vi "Main Monitor Loop.vi"(8 "error in (no error)":errorcluster, 11 "main ref":T1) -> (0 "error out":errorcluster)   [LabVIEW 2025]
uses:
  controls/LAB-IQ UI Data.ctl
panel:
  out "Test Stop Temp":bool
  out "DepthZ":dbl
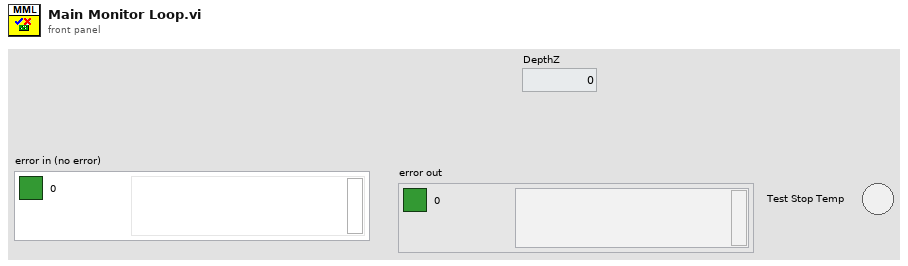
[diagram p1: front panel]
types:
  T1 = typedef "LAB-IQ UI Data.ctl" = cluster{"Main Home Screen":cluster{"GUI":refnum<vi>, "Platform Settings":refnum<vi>, "Configure":refnum<vi>, "Home":refnum<vi>, "EXIT":refnum<vi>, "service 2":refnum<vi>, "MainPage":refnum<vi>, "Analysis":refnum<vi>}, "Platform Settings":cluster{"mm/s  Surge":refnum<vi>, "Update Surge Speed":refnum<vi>, "Drive Error":refnum<vi>, "Disable Axis Jog Soft Limits":refnum<vi>, "mm/s  Sway":refnum<vi>, "Sway and Surge COM Status":refnum<vi>, "Heave COM Status":refnum<vi>, "Enable Platform":refnum<vi>, "Surge Forward Main":refnum<vi>, "Sway Right Main":refnum<vi>, "Sway Left Main":refnum<vi>, "Heave Down Main":refnum<vi>, "Heave Up main":refnum<vi>, "Update Sway Speed":refnum<vi>, "Update Heave Speed":refnum<vi>, "mm/s Heave":refnum<vi>, "mm/sec":refnum<vi>, "mm":refnum<vi>, "Surge Backward Main":refnum<vi>}, "Analysis Screen":cluster{"Analysis Home":refnum<vi>, "Surface Analysis":refnum<vi>, "Imaging":refnum<vi>, "Image Analysis":refnum<vi>, "Post Analysis":refnum<vi>}, "Config Screen":cluster{"Select Load Head":refnum<vi>, "Notes :":refnum<vi>, "FILE":refnum<vi>, "Sample ID :":refnum<vi>, "Operator ID :":refnum<vi>, "Operator Name :":refnum<vi>, "Auto":refnum<vi>}, "Motion Module":cluster{"zNL":refnum<vi>, "NL disp":refnum<vi>, "Rotary Tab":refnum<vi>, "Motion Direction:  3":refnum<vi>, "E.Velocity 2":refnum<vi>, "e.v/ssr 2":refnum<vi>, "Enter Fixed E.Velocity 2":refnum<vi>, "Enter Final SRR 2":refnum<vi>, "Enter initial SRR 2":refnum<vi>, "Enter Fixed SRR 2":refnum<vi>, "Enter the Final E.Velocity (m/s) 2":refnum<vi>, "Enter initial E.Velocity (m/s) 2":refnum<vi>, "Final Speed (RPM) 3":refnum<vi>, "Initial Speed (RPM) 2":refnum<vi>, "Enter the Final Velocity (m/s) 3":refnum<vi>, "Enter initial Velocity (m/s)  3":refnum<vi>, "Ramp Up 2":refnum<vi>, "TEST SELECTION":refnum<vi>, "SPEED SELECTION : ":refnum<vi>, "Angular Oscillation Set":refnum<vi>, "Traction":refnum<vi>, "Step Speed":refnum<vi>, "StepTable For Load-Speed":refnum<vi>, "StepTable For Speed":refnum<vi>, "Surge Forward MM":refnum<vi>, "Surge Backward MM":refnum<vi>, "M3 Image":refnum<vi>, "String 39":refnum<vi>, "Sway Left MM":refnum<vi>, "Sway Right MM":refnum<vi>, "Disable Axis Jog Soft Limits":refnum<vi>, "mm":refnum<vi>, "Heave Down MM":refnum<vi>, "Heave Up MM":refnum<vi>, "Wear Track Diameter (mm)":refnum<vi>, "Set WTD":refnum<vi>, "HomeScratch":refnum<vi>, "HomeRot":refnum<vi>, "PlaceModule":refnum<vi>, "Enter the Angle (Deg)":refnum<vi>, "Enter the Frequency (Hz)":refnum<vi>, "Motion Mode:":refnum<vi>, "LR Sway":refnum<vi>, "Rot Hor":refnum<vi>, "Scratch":refnum<vi>, "LR Cam":refnum<vi>, "MMBack":refnum<vi>, "MMNext":refnum<vi>, "Rot Ver":refnum<vi>, "Rotary Module Selection":refnum<vi>, "calculate rotary":refnum<vi>, "SPEED SELECTION : rotary":refnum<vi>, "Import 2":refnum<vi>, "Save 2":refnum<vi>, "File Path :  2":refnum<vi>, "String 45":refnum<vi>, "StepTable For Speed 3":refnum<vi>, "Enter the Speed(mm/sec)":refnum<vi>, "Enter the Speed(RPM)":refnum<vi>, "Enter Scratch Speed (mm/s):":refnum<vi>, "SwaySpeed Set":refnum<vi>, "Scartch Offset":refnum<vi>, "Motion type:":refnum<vi>, "HomeScratch 2":refnum<vi>, "Enter Scratch length (mm):":refnum<vi>, "Wear Track Diameter":refnum<vi>, "Rotary Speed Exced":refnum<vi>, "Scratch Mode":refnum<vi>, "No of Scratch":refnum<vi>}, "Environmental control":cluster{"Humidity  Status  3":refnum<vi>, "Low Temp  Status  2":refnum<vi>, "TK4 status 2":refnum<vi>, "Stage Temperature":refnum<vi>, "Sample Temperature":refnum<vi>, "Humidity (Amb)":refnum<vi>, "Clear List":refnum<vi>, "Add to list":refnum<vi>, "Wear":refnum<vi>, "Vibration":refnum<vi>, "Humidity (Chamber)":refnum<vi>, "Temperature (Chamber)":refnum<vi>, "ECR ":refnum<vi>, "Temperature (Amb)":refnum<vi>, "Microphone":refnum<vi>, "Acoustic Emission 3":refnum<vi>, "SNext":refnum<vi>, "APBack":refnum<vi>, "Enter the Temperature (°C):":refnum<vi>, "Enter the Stage \nTemperature (°C):":refnum<vi>, "Enter the Humidity (%Rh):":refnum<vi>, "Low Temp":refnum<vi>, "High Temp":refnum<vi>, "Humidity":refnum<vi>, "Sensors Picked":refnum<vi>}, "About Screen":cluster{"Password":refnum<vi>, "Home Service":refnum<vi>, "Advanced Setting":refnum<vi>, "About Tab":refnum<vi>, "ECR Port:":refnum<vi>, "Ramp Port:":refnum<vi>, "Installation/Replacement completed":refnum<vi>, "Loahead":refnum<vi>, "Heave and Surge COM Port:":refnum<vi>, "Sway COM Port:":refnum<vi>, "Temp Modbus:":refnum<vi>, "Humidity Port:":refnum<vi>, "Edit Gain Constants":refnum<vi>, "Save Gain Constants":refnum<vi>}, "Main Screen":cluster{"Main Screen Tab":refnum<vi>, "Angle and Frequency":refnum<vi>, "Stroke (mm)":refnum<vi>, "Angle (Deg)":refnum<vi>, "Main Speed Tab":refnum<vi>, "MTM MOTOR DISPLAY":refnum<vi>, "Disc Speed (m/sec)":refnum<vi>, "Ball Speed (m/sec)":refnum<vi>, "Disc Speed (RPM)":refnum<vi>, "Ball Speed (RPM)":refnum<vi>, "SPEED TAB":refnum<vi>, "Speed (m/sec)":refnum<vi>, "Set Speed (m/sec)":refnum<vi>, "Speed (RPM)":refnum<vi>, "Set Speed":refnum<vi>, "Time Tab":refnum<vi>, "Time ( HH:MM:SS ) 2":refnum<vi>, "Test Duration":refnum<vi>, "Test Duration 4":refnum<vi>, "TEST CYCLE":refnum<vi>, "TOTAL CYCLES":refnum<vi>, "Set Load (N)":refnum<vi>, "Temp Tabs":refnum<vi>, "Heater":refnum<vi>, "TK4 status":refnum<vi>, "ChamberTemp":refnum<vi>, "SetTmp":refnum<vi>, "Controller  Status":refnum<vi>, "ChamberTemp 2":refnum<vi>, "SetTmp 2":refnum<vi>, "Controller  Status 2":refnum<vi>, "ChamberTemp 3":refnum<vi>, "SetTmp 3":refnum<vi>, "Cooling":refnum<vi>, "Load Communication":refnum<vi>, "Ambient \nTemperature":refnum<vi>, "HumCOMStatus":refnum<vi>, "Ambient\n Humidity":refnum<vi>, "Freq (Hz)":refnum<vi>, "Load En":refnum<vi>, "NLt":refnum<vi>, "zNL 2":refnum<vi>, "Humidity On":refnum<vi>, "humidity disp":refnum<vi>, "Set Humidity":refnum<vi>, "NL disp 2":refnum<vi>, "Humidity On 2":refnum<vi>, "humidity disp 2":refnum<vi>, "Set Humidity 2":refnum<vi>, "NL disp 3":refnum<vi>, "AppLoadSeq scratch":refnum<vi>, "Stop Scratch":refnum<vi>, "ClrLog":refnum<vi>, "Trip Log":refnum<vi>, "STOP":refnum<vi>, "Start Test":refnum<vi>, "Test status":refnum<vi>, "AR Led":refnum<vi>, "Data":refnum<vi>, "Health":refnum<vi>, "Sway COM Status":refnum<vi>, "Heave COM Status":refnum<vi>, "Grp Tab":refnum<vi>, "Sub Graph":refnum<vi>, "SD (mm)":refnum<vi>, "Siliding distance Reset Graph":refnum<vi>, "SDGp":refnum<vi>, "Humidity Reset Graph":refnum<vi>, "HumrGp":refnum<vi>, "Acoustic Emission (mV)":refnum<vi>, "Aqucostic Reset Graph":refnum<vi>, "gACQUOS":refnum<vi>, "ECR RESET":refnum<vi>, "ECR":refnum<vi>, "Temperature Reset":refnum<vi>, "Acoustic Emission (mV) 2":refnum<vi>, "Aqucostic Reset Graph 2":refnum<vi>, "gACQUOS 2":refnum<vi>, "ECR RESET 2":refnum<vi>, "ECR 2":refnum<vi>, "Temperature Reset 2":refnum<vi>, "Temperature (deg c)":refnum<vi>, "Speed Reset Graph":refnum<vi>, "Speed Tab":refnum<vi>, "MTM DISC  SPEED":refnum<vi>, "MTM BALL SPEED":refnum<vi>, "speed mm/sec":refnum<vi>, "Hymidity":refnum<vi>, "Humidity Disable trip":refnum<vi>, "CoF Trip  2":refnum<vi>, "Depth Trip":refnum<vi>, "Weart Deapth":refnum<vi>, "Depth Reset Graph":refnum<vi>, "Weart":refnum<vi>, "Depthz":refnum<vi>, "Depth (µm)":refnum<vi>, "WearGp":refnum<vi>, "NL Trip 2":refnum<vi>, "Load pid":refnum<vi>, "Load Disable Trip":refnum<vi>, "Load Reset Graph":refnum<vi>, "NL Display 4":refnum<vi>, "Main Chart 3":refnum<vi>, "BACK":refnum<vi>, "Depth Trip 2":refnum<vi>, "COF TRIP ":refnum<vi>, "Friction Force (N)":refnum<vi>, "FF Reset Graph":refnum<vi>, "FF Disable Trip":refnum<vi>, "FF TRIP":refnum<vi>, "COF Disable Trip":refnum<vi>, "COF Reset Graph":refnum<vi>, "Start Test Temp":refnum<vi>, "zFF":refnum<vi>, "Friction Force (N) Graph":refnum<vi>, "Coefficient of Friction":refnum<vi>, "Scratch Start Test":refnum<vi>, "FF Tab":refnum<vi>, "Cyclic Friction Force (N)":refnum<vi>, "CZ FF":refnum<vi>, "Cyclic Friction Force (N) Graph":refnum<vi>, "Cyclic Coefficient of Friction":refnum<vi>, "Cyclic FF TRIP":refnum<vi>, "Cyclic FF Disable Trip":refnum<vi>, "cyclic COF Disable Trip":refnum<vi>, "cyclic COF TRIP":refnum<vi>, "cyclic COF Reset Graph":refnum<vi>, "Cyclic FF Reset Graph":refnum<vi>, "Test Trip":refnum<vi>, "Multi Scratch Pass":refnum<vi>, "Scratch Start Recording":refnum<vi>}, "Loading":cluster{"Indentation":refnum<vi>, "Reference Sample":refnum<vi>, "Load Cell Communication Slide":refnum<vi>, "com 3":refnum<vi>, "com":refnum<vi>, "DecaForce COM Status":refnum<vi>, "Update":refnum<vi>, "Clear 3":refnum<vi>, "seq":refnum<vi>, "Stribeck table":refnum<vi>, "Stribeck Table  For loading":refnum<vi>, "Loading Mode":refnum<vi>, "Enter the Final Load (N)":refnum<vi>, "Enter the CoF Trip":refnum<vi>, "Enter the Friction Force Trip":refnum<vi>, "Enter the Normal load Trip":refnum<vi>, "Enter the Load  (N)":refnum<vi>, "KiloForce":refnum<vi>, "DecaForce ":refnum<vi>, "MicroForce":refnum<vi>, "LHBack":refnum<vi>, "LHNext":refnum<vi>, "Enter the Loading Rate (N/min)":refnum<vi>, "Message":refnum<vi>, "Warning 2":refnum<vi>, "SSP 0.75":refnum<vi>, "SSP 0.5":refnum<vi>, "SSP 0.3":refnum<vi>, "Warning":refnum<vi>, "gui GIF":refnum<vi>, "Communication is established":refnum<vi>, "AppLoad 4":refnum<vi>, "Multipoint":refnum<vi>, "Load Selection":refnum<vi>}, "PID":cluster{"Ramp MulFac":refnum<vi>, "pulses LoadDiffRamp(2..10)":refnum<vi>, "PulseControlRamp(diff<=3N)":refnum<vi>, "SetLoadDeadband(%) Load(0-10N)":refnum<vi>, "PID gains out delay (microForce)":refnum<vi>, "Ramp":refnum<vi>, "Gain 2":refnum<vi>, "pulses LoadDiff(2..10)":refnum<vi>, "pulses LoadDiff(11..50)":refnum<vi>, "PulseControl(diff<=3N)":refnum<vi>, "SetLoadDeadband(%)  2":refnum<vi>, "Dummy Run":refnum<vi>, "Vertical load (N)":refnum<vi>, "AutoTune":refnum<vi>, "Offset 3 ":refnum<vi>, "apply load":refnum<vi>, "Offset  3":refnum<vi>, "apply load 2":refnum<vi>, "Enter ByPass Load":refnum<vi>, "reinit 3":refnum<vi>, "output range delay":refnum<vi>, "PID gains out delay":refnum<vi>, "Bypass Load":refnum<vi>, "pulsesSent":refnum<vi>, "pulses ":refnum<vi>, "actpid":refnum<vi>, "gFF Rot":refnum<vi>, "pulses LoadDiff(21..1000)":refnum<vi>, "Delay":refnum<vi>, "deadband":refnum<vi>}, "Config Parameters":cluster{"Tab Control 3":refnum<vi>, "Tab Control 19":refnum<vi>, "SAMPLES":refnum<vi>, "Re-initilaize":refnum<vi>, "Filter ON/OFF":refnum<vi>, "TracHomeSurgeOffsetCounts 10MM":refnum<vi>, "TracHomeSwayOffsetCounts 10MM":refnum<vi>, "Acoustic Emission:":refnum<vi>, "Apply Filter (FF)":refnum<vi>, "Filter% 2":refnum<vi>, "Apply Filter (Load)":refnum<vi>, "Filter% ":refnum<vi>, "Sway distance (mm)":refnum<vi>, "Surge distance (mm)":refnum<vi>, "DataSavingLoopDelay(ms)":refnum<vi>, "SAVE 2":refnum<vi>, "Enter Distance":refnum<vi>, "Sway Counts:":refnum<vi>, "Distance (mm): 3":refnum<vi>, "Surge Counts:":refnum<vi>, "Distance (mm): 2":refnum<vi>, "Distance (mm):":refnum<vi>, "Heave Counts:":refnum<vi>, "LRMHomeSurgeOffsetCounts":refnum<vi>, "LRMHomeSwayOffsetCounts":refnum<vi>, "TracHomeSurgeOffsetCounts 20MM":refnum<vi>, "TracHomeSwayOffsetCounts 20MM":refnum<vi>, "RotHomeSwayOffsetCounts":refnum<vi>, "RotHomeSurgeOffsetCounts":refnum<vi>, "Heave distance":refnum<vi>, "Zmm":refnum<vi>, "Heave Pulses/mm":refnum<vi>, "Surge Pulses/mm":refnum<vi>, "Sway Pulses/mm":refnum<vi>, "Heave Pitch":refnum<vi>, "Surge Pitch":refnum<vi>, "Sway Pitch":refnum<vi>, "Heave PPR":refnum<vi>, "Surge PPR":refnum<vi>, "Sway PPR":refnum<vi>, "Tab Control 5":refnum<vi>, "Tab Control 14":refnum<vi>, "Tab Control 26":refnum<vi>, "AE":refnum<vi>, "Heave Loop Delay":refnum<vi>, "Heave PID Speed":refnum<vi>, "Surge Jog Speed":refnum<vi>, "Heave Jog Speed":refnum<vi>, "Sway Loop Delay":refnum<vi>, "Sway PID Speed":refnum<vi>, "Sway Jog Speed":refnum<vi>, "DEPTH TRIP VALUE":refnum<vi>, "LOAD TRIP VALUE":refnum<vi>, "DEPTH TRIP   ENABLE":refnum<vi>, "LOAD TRIP  ENABLE":refnum<vi>, "CYCLIC FF TRIP VALUE":refnum<vi>, "FF TRIP VALUE":refnum<vi>, "CYCLIC CoF TRIP VALUE":refnum<vi>, "COF TRIP VALUE":refnum<vi>, "CYCLIC COF TRIP  ENABLE":refnum<vi>, "CYCLIC FF TRIP  ENABLE":refnum<vi>, "FF TRIP  ENABLE":refnum<vi>, "COF TRIP  ENABLE":refnum<vi>}, "Loading Com Port":cluster{"ClearAll":refnum<vi>, "Mz(Nm)":refnum<vi>, "My(Nm)":refnum<vi>, "Mx(Nm)":refnum<vi>, "Save Dwell":refnum<vi>, "Mx ":refnum<vi>, "My ":refnum<vi>, "Mz":refnum<vi>, "Fx(N)":refnum<vi>, "Fy(N)":refnum<vi>, "Fz(N)":refnum<vi>, "ZeroAll":refnum<vi>, "Acq Delay (ms)":refnum<vi>, "Burst Delay (ms)":refnum<vi>, "model":refnum<vi>, "SN":refnum<vi>, "FFx(N)":refnum<vi>, "Sensor IP":refnum<vi>, "Port":refnum<vi>, "FFy(N)":refnum<vi>, "Load(N)":refnum<vi>, "delete Handle":refnum<vi>, "Create Handle":refnum<vi>, "ft_data":refnum<vi>, "ft_range":refnum<vi>, "ft_data 2":refnum<vi>, "stop 6":refnum<vi>, "running_flag":refnum<vi>, "ft_udp_handle":refnum<vi>, "get-data-return":refnum<vi>, "get-range-return":refnum<vi>, "zero-return":refnum<vi>, "filter-return":refnum<vi>, "initial-return":refnum<vi>, "deleteHandle-result":refnum<vi>, "Load Cell Temp":refnum<vi>}, "Heave AND Surge":cluster{"SURGE POSE":refnum<vi>, "error out Read":refnum<vi>, "HEAVE POSE":refnum<vi>, "State":refnum<vi>, "Homed":refnum<vi>, "Sequence ID":refnum<vi>, "error out Write":refnum<vi>, "faultCode":refnum<vi>, "Ack ID":refnum<vi>, "SPEED":refnum<vi>, "Distance":refnum<vi>, "Mode Command":refnum<vi>, "Heave and Surge Read":refnum<vi>, "Read Heave Temp":refnum<vi>, "Spare 15":refnum<vi>, "Spare 14":refnum<vi>, "Spare 13":refnum<vi>, "Spare 12":refnum<vi>, "Spare 11":refnum<vi>, "Spare 10":refnum<vi>, "Spare 9":refnum<vi>, "Spare 8":refnum<vi>, "Spare 7":refnum<vi>, "Spare 6":refnum<vi>, "Spare 5":refnum<vi>, "Spare 4":refnum<vi>, "Spare 2":refnum<vi>, "Spare 1":refnum<vi>, "Node Id":refnum<vi>, "Spare 3":refnum<vi>, "SPARE 4":refnum<vi>, "SPARE 3":refnum<vi>, "SPARE 2":refnum<vi>, "SPARE 1":refnum<vi>, "fwMajor":refnum<vi>, "fwMinor":refnum<vi>, "Manual Write":refnum<vi>, "Heave and Surge Write":refnum<vi>}, "New PID LOGIC":cluster{"Fine Tune Zone":refnum<vi>, "PID SDelay":refnum<vi>, "Max_pos_limit":refnum<vi>, "Min_pos_limit":refnum<vi>, "i_limit":refnum<vi>, "pct_scale":refnum<vi>, "Deadband":refnum<vi>, "Kd":refnum<vi>, "Ki":refnum<vi>, "Kp":refnum<vi>, "Current Position":refnum<vi>, "Set Load":refnum<vi>, "Current Load":refnum<vi>, "Pulse delta":refnum<vi>, "Init Step":refnum<vi>, "Max Step Linit":refnum<vi>}, "SWAY ":cluster{"fwMajor":refnum<vi>, "Homed":refnum<vi>, "Rotary POSE":refnum<vi>, "State":refnum<vi>, "SWAY POSE":refnum<vi>, "Ack ID":refnum<vi>, "faultCode":refnum<vi>, "Node Id":refnum<vi>, "fwMinor":refnum<vi>, "Spare 6":refnum<vi>, "Spare 5":refnum<vi>, "Spare 4":refnum<vi>, "Spare 3":refnum<vi>, "Spare 2":refnum<vi>, "Spare 1":refnum<vi>, "Spare 7":refnum<vi>, "SPARE  5":refnum<vi>, "error out Write  SWAY ":refnum<vi>, "error out Read SWAY ":refnum<vi>, "Manual Write SWAY ":refnum<vi>, "SWAY WRITE":refnum<vi>, "SPARE  4":refnum<vi>, "SPARE  3":refnum<vi>, "SPARE 2":refnum<vi>, "SPARE 1":refnum<vi>, "Spare 15":refnum<vi>, "Spare 14":refnum<vi>, "Spare 13":refnum<vi>, "Spare 12":refnum<vi>, "Spare 11":refnum<vi>, "Spare 9":refnum<vi>, "Spare 8":refnum<vi>, "SPEED":refnum<vi>, "Distance":refnum<vi>, "Mode Command":refnum<vi>, "Sequence ID":refnum<vi>, "SWAY READ":refnum<vi>, "Spare 10":refnum<vi>, "Read SWAY Temp":refnum<vi>}, "Analysis Screen":cluster{"Analysis Home":refnum<vi>, "Refresh 2":refnum<vi>, "MEAN 4":refnum<vi>, "SD 4":refnum<vi>, "VARIANCE 4":refnum<vi>, "MEAN  3":refnum<vi>, "SD  3":refnum<vi>, "VARIANCE  3":refnum<vi>, "MEAN 2":refnum<vi>, "SD  2":refnum<vi>, "VARIANCE 2":refnum<vi>, "MEAN":refnum<vi>, "SD":refnum<vi>, "VARIANCE":refnum<vi>, "File 4 Discription":refnum<vi>, "OPEN 4":refnum<vi>, "File Name 4":refnum<vi>, "OPEN 3":refnum<vi>, "File 3 Discription":refnum<vi>, "File Name 3":refnum<vi>, "Y-AXIS":refnum<vi>, "X-AXIS":refnum<vi>, "XY Graph":refnum<vi>, "File Name 2":refnum<vi>, "File Name 1":refnum<vi>, "OPEN 2":refnum<vi>, "OPEN 1":refnum<vi>, "File 1 Discription ":refnum<vi>, "File 2 Discription":refnum<vi>, "Export":refnum<vi>, "File Format":refnum<vi>}}
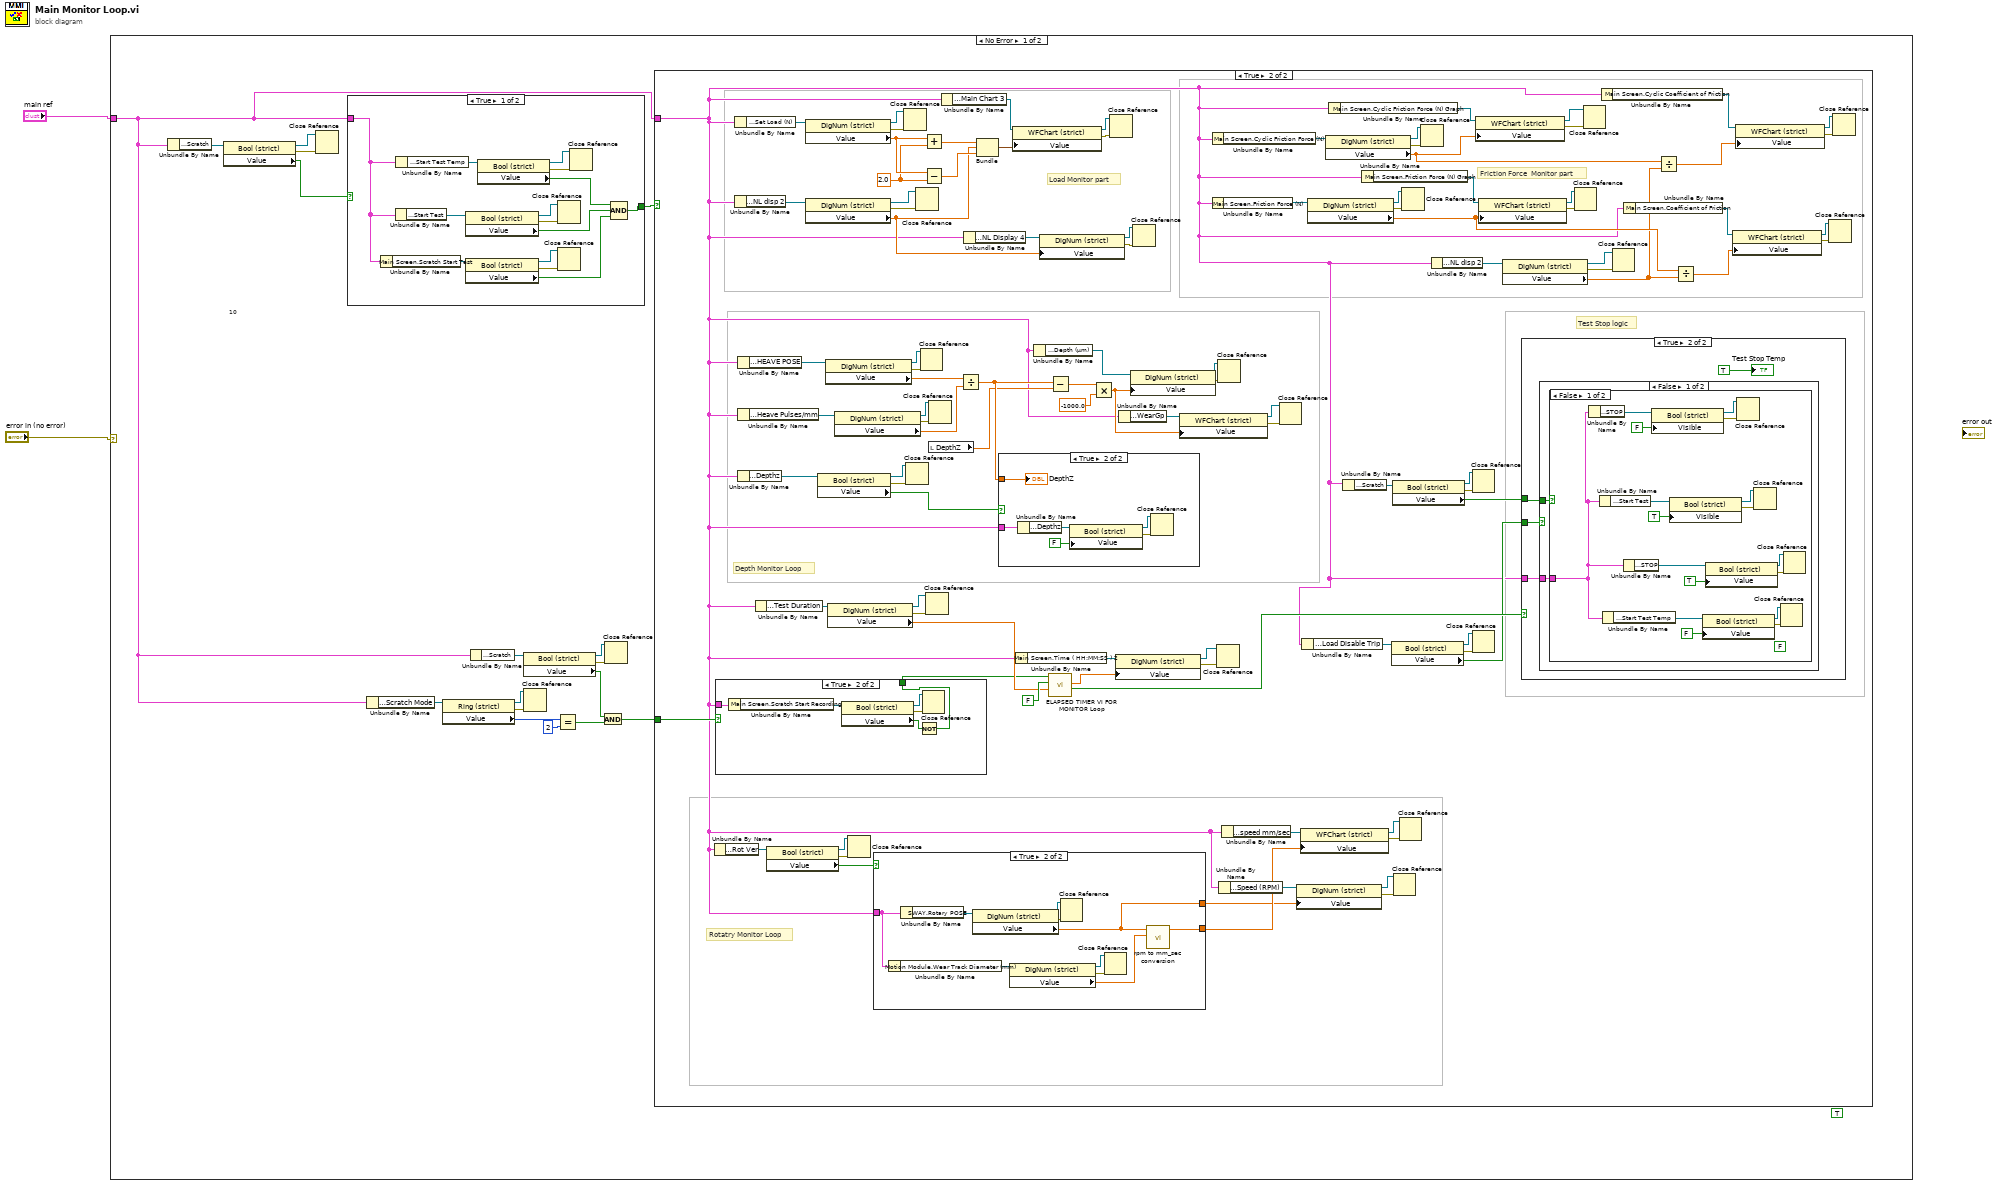
[diagram p0: block diagram]
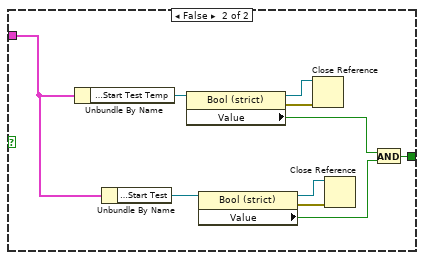
[diagram p2: hidden frame]
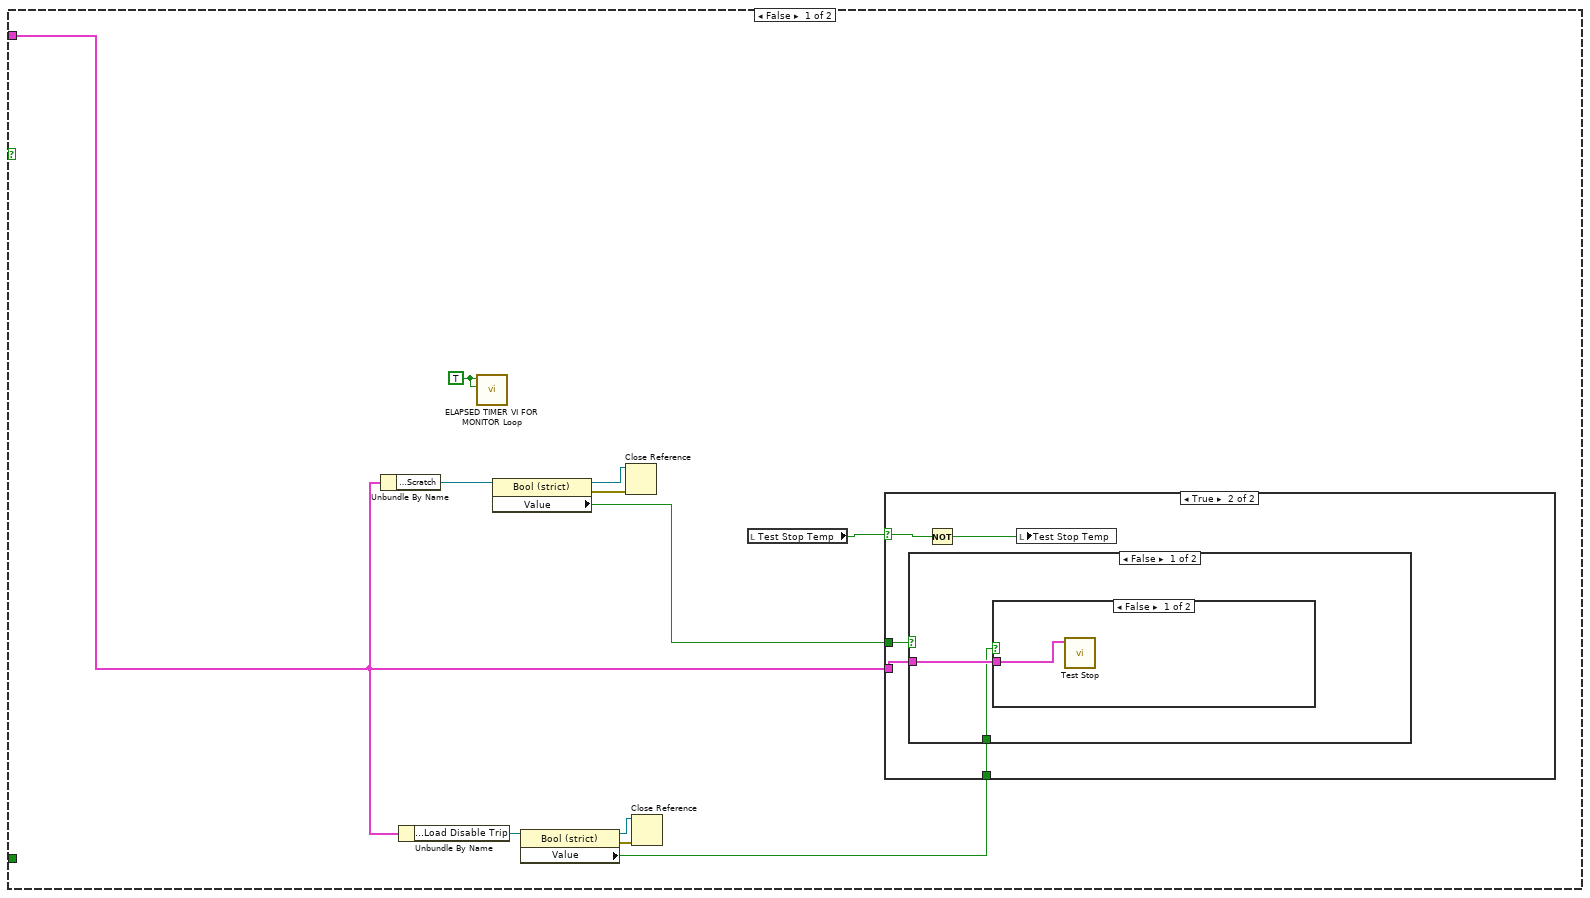
[diagram p3: hidden frame]
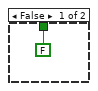
[diagram p7: hidden frame]
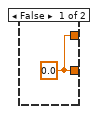
[diagram p8: hidden frame]
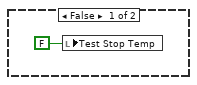
[diagram p9: hidden frame]
diagram:
  n1 = case shown="No Error" "error in (no error)" {
    tunnel: "main ref" -> [w6 _]
    frame No Error {
      (unwired) TRUE
      # "10"
      n2 = Unbundle By Name(w6) -> ("Motion Module.Scratch"=w17:refnum<vi>)
      n3 = property class="Bool (strict)"(reference=w17) -> (reference out=w18:refnum<vi>, error out=w16:errorcluster, "Value"=w15:bool)  [unwired: 1 in]
      n4 = Close Reference(reference=w18, error in (no error)=w16) -> ()  [unwired: 1 out]
      n5 = case shown="True" w15 {
        tunnel: w6 -> [w21 w37]
        tunnel: [w25 w35] -> w19
        frame True {
          n6 = Unbundle By Name(w21) -> ("Main Screen.Scratch Start Test"=w23:refnum<vi>)
          n7 = Unbundle By Name(w21) -> ("Main Screen.Start Test"=w29:refnum<vi>)
          n8 = Unbundle By Name(w21) -> ("Main Screen.Start Test Temp"=w32:refnum<vi>)
          n9 = property class="Bool (strict)"(reference=w29) -> (reference out=w28:refnum<vi>, error out=w30:errorcluster, "Value"=w26:bool)  [unwired: 1 in]
          n10 = property class="Bool (strict)"(reference=w23) -> (reference out=w24:refnum<vi>, error out=w22:errorcluster, "Value"=w20:bool)  [unwired: 1 in]
          n11 = property class="Bool (strict)"(reference=w32) -> (reference out=w33:refnum<vi>, error out=w31:errorcluster, "Value"=w27:bool)  [unwired: 1 in]
          n12 = Close Reference(reference=w28, error in (no error)=w30) -> ()  [unwired: 1 out]
          n13 = Close Reference(reference=w24, error in (no error)=w22) -> ()  [unwired: 1 out]
          n14 = Close Reference(reference=w33, error in (no error)=w31) -> ()  [unwired: 1 out]
          n15 = Compound Arithmetic op=AND(w27, w26, w20) -> (w25:bool)
        }
        frame False {
          n16 = Unbundle By Name(w37) -> ("Main Screen.Start Test Temp"=w42:refnum<vi>)
          n17 = Unbundle By Name(w37) -> ("Main Screen.Start Test"=w39:refnum<vi>)
          n18 = property class="Bool (strict)"(reference=w42) -> (reference out=w43:refnum<vi>, error out=w41:errorcluster, "Value"=w36:bool)  [unwired: 1 in]
          n19 = property class="Bool (strict)"(reference=w39) -> (reference out=w38:refnum<vi>, error out=w40:errorcluster, "Value"=w34:bool)  [unwired: 1 in]
          n20 = Close Reference(reference=w43, error in (no error)=w41) -> ()  [unwired: 1 out]
          n21 = Close Reference(reference=w38, error in (no error)=w40) -> ()  [unwired: 1 out]
          n22 = And(x=w36, y=w34) -> (x .and. y?=w35:bool)
        }
      }
      n23 = Unbundle By Name(w6) -> ("Motion Module.Scratch Mode"=w10:refnum<vi>)
      n24 = property class="Ring (strict)"(reference=w10) -> (reference out=w11:refnum<vi>, error out=w9:errorcluster, "Value"=w8:u16)  [unwired: 1 in]
      n25 = Unbundle By Name(w6) -> ("Motion Module.Scratch"=w13:refnum<vi>)
      n26 = property class="Bool (strict)"(reference=w13) -> (reference out=w12:refnum<vi>, error out=w14:errorcluster, "Value"=w4:bool)  [unwired: 1 in]
      n27 = Close Reference(reference=w11, error in (no error)=w9) -> ()  [unwired: 1 out]
      n28 = Equal?(x=w8, y=u16 2) -> (x = y?=w5:bool)
      n29 = And(x=w4, y=w5) -> (x .and. y?=w3:bool)
      n30 = Close Reference(reference=w12, error in (no error)=w14) -> ()  [unwired: 1 out]
      n31 = case shown="True" w19 {
        tunnel: w6 -> [w45 w64]
        tunnel: w3 -> [_ w65]
        frame False {
          w54 = TRUE ("PAUSE")
          n32 = Unbundle By Name(w45) -> ("Motion Module.Scratch"=w52:refnum<vi>)
          n33 = Unbundle By Name(w45) -> ("Main Screen.Load Disable Trip"=w46:refnum<vi>)
          n34 = call "ELAPSED TIMER VI FOR MONITOR Loop.vi"("RESET"=w54, "PAUSE"=w54) -> ()  [unwired: 7 in, 3 out]
          n35 = property class="Bool (strict)"(reference=w52) -> (reference out=w50:refnum<vi>, error out=w51:errorcluster, "Value"=w49:bool)  [unwired: 1 in]
          n36 = property class="Bool (strict)"(reference=w46) -> (reference out=w48:refnum<vi>, error out=w47:errorcluster, "Value"=w44:bool)  [unwired: 1 in]
          n37 = Close Reference(reference=w50, error in (no error)=w51) -> ()  [unwired: 1 out]
          n38 = Close Reference(reference=w48, error in (no error)=w47) -> ()  [unwired: 1 out]
          n39 = local read "Test Stop Temp"() -> (w53:bool)
          n40 = case shown="True" w53 {
            selector: w53 -> [_ w59]
            tunnel: w45 -> [_ w57]
            tunnel: w49 -> [_ w56]
            tunnel: w44 -> [_ w55]
            frame False {
            }
            frame True {
              n41 = case shown="False" w56 {
                tunnel: w57 -> [w61 _]
                tunnel: w55 -> [w60 _]
                frame False {
                  n42 = case shown="False" w60 {
                    tunnel: w61 -> [w62 _]
                    frame False {
                      n43 = call "Test Stop.vi"("Data Cluster"=w62) -> ()  [unwired: 10 in, 1 out]
                    }
                    frame True {
                    }
                  }
                }
                frame True {
                }
              }
              n44 = Not(x=w59) -> (.not. x?=w58:bool)
              n45 = local write "Test Stop Temp"(w58) -> ()
            }
          }
        }
        frame True {
          w150 = 2.0 ("y")
          # "Rotatry Monitor Loop"
          # "Test Stop logic"
          # "Depth Monitor Loop"
          # "Friction Force  Monitor part"
          # "Load Monitor part"
          n46 = Unbundle By Name(w64) -> ("Motion Module.Rot Ver"=w81:refnum<vi>)
          n47 = case shown="True" w65 {
            tunnel: w64 -> [_ w166]
            tunnel: [FALSE ("Value") w164] -> w63
            frame False {
            }
            frame True {
              n48 = Unbundle By Name(w166) -> ("Main Screen.Scratch Start Recording"=w168:refnum<vi>)
              n49 = property class="Bool (strict)"(reference=w168) -> (reference out=w167:refnum<vi>, error out=w169:errorcluster, "Value"=w165:bool)  [unwired: 1 in]
              n50 = Not(x=w165) -> (.not. x?=w164:bool)
              n51 = Close Reference(reference=w167, error in (no error)=w169) -> ()  [unwired: 1 out]
            }
          }
          n52 = Unbundle By Name(w64) -> ("Main Screen.Set Load (N)"=w152:refnum<vi>)
          n53 = Unbundle By Name(w64) -> ("Main Screen.NL disp 2"=w162:refnum<vi>)
          n54 = Unbundle By Name(w64) -> ("Heave AND Surge.HEAVE POSE"=w144:refnum<vi>)
          n55 = Unbundle By Name(w64) -> ("Config Parameters.Heave Pulses/mm"=w141:refnum<vi>)
          n56 = Unbundle By Name(w64) -> ("Main Screen.Depthz"=w136:refnum<vi>)
          n57 = Unbundle By Name(w64) -> ("Main Screen.Test Duration"=w120:refnum<vi>)
          n58 = property class="Bool (strict)"(reference=w81) -> (reference out=w79:refnum<vi>, error out=w80:errorcluster, "Value"=w78:bool)  [unwired: 1 in]
          n59 = property class="DigNum (strict)"(reference=w152) -> (reference out=w146:refnum<vi>, error out=w153:errorcluster, "Value"=w151:dbl)  [unwired: 1 in]
          n60 = property class="DigNum (strict)"(reference=w162) -> (reference out=w160:refnum<vi>, error out=w161:errorcluster, "Value"=w97:dbl)  [unwired: 1 in]
          n61 = property class="Bool (strict)"(reference=w136) -> (reference out=w137:refnum<vi>, error out=w135:errorcluster, "Value"=w134:bool)  [unwired: 1 in]
          n62 = property class="DigNum (strict)"(reference=w144) -> (reference out=w145:refnum<vi>, error out=w143:errorcluster, "Value"=w139:sgl)  [unwired: 1 in]
          n63 = property class="DigNum (strict)"(reference=w120) -> (reference out=w121:refnum<vi>, error out=w119:errorcluster, "Value"=w118:dbl)  [unwired: 1 in]
          n64 = property class="DigNum (strict)"(reference=w141) -> (reference out=w140:refnum<vi>, error out=w142:errorcluster, "Value"=w138:dbl)  [unwired: 1 in]
          n65 = Close Reference(reference=w79, error in (no error)=w80) -> ()  [unwired: 1 out]
          n66 = case shown="True" w78 {
            tunnel: w64 -> [_ w174]
            tunnel: [w170 w172] -> w74
            tunnel: [w170 w171] -> w70
            frame False {
              w170 = 0.0 ("Enter initial Velocity (m/s)  4")
            }
            frame True {
              n67 = Unbundle By Name(w174) -> ("Motion Module.Wear Track Diameter (mm)"=w177:refnum<vi>)
              n68 = Unbundle By Name(w174) -> ("SWAY.Rotary POSE"=w178:refnum<vi>)
              n69 = property class="DigNum (strict)"(reference=w178) -> (reference out=w180:refnum<vi>, error out=w179:errorcluster, "Value"=w171:sgl)  [unwired: 1 in]
              n70 = property class="DigNum (strict)"(reference=w177) -> (reference out=w175:refnum<vi>, error out=w176:errorcluster, "Value"=w173:dbl)  [unwired: 1 in]
              n71 = Close Reference(reference=w180, error in (no error)=w179) -> ()  [unwired: 1 out]
              n72 = Close Reference(reference=w175, error in (no error)=w176) -> ()  [unwired: 1 out]
              n73 = call "rpm to mm_sec conversion.vi"("Wear Track Diameter"=w173, "Initial Speed (RPM)"=w171) -> ("Enter initial Velocity (m/s)  4"=w172:dbl)  [unwired: 7 in, 2 out]
            }
          }
          n74 = Close Reference(reference=w146, error in (no error)=w153) -> ()  [unwired: 1 out]
          n75 = Close Reference(reference=w137, error in (no error)=w135) -> ()  [unwired: 1 out]
          n76 = Close Reference(reference=w160, error in (no error)=w161) -> ()  [unwired: 1 out]
          n77 = Close Reference(reference=w145, error in (no error)=w143) -> ()  [unwired: 1 out]
          n78 = Add(x=w151, y=w150) -> (x+y=w149:dbl)
          n79 = Subtract(x=w151, y=w150) -> (x-y=w148:dbl)
          n80 = Close Reference(reference=w121, error in (no error)=w119) -> ()  [unwired: 1 out]
          n81 = Close Reference(reference=w140, error in (no error)=w142) -> ()  [unwired: 1 out]
          n82 = local read "DepthZ"() -> (w132:dbl)
          n83 = Unbundle By Name(w64) -> ("Main Screen.Main Chart 3"=w156:refnum<vi>)
          n84 = Divide(x=w139, y=w138) -> (x/y=w133:dbl)
          n85 = Unbundle By Name(w64) -> ("Main Screen.NL Display 4"=w157:refnum<vi>)
          n86 = Bundle(w149, "Value"=w97, w148) -> (w147:cluster{dbl, "Value":dbl, dbl})  [unwired: 1 in]
          n87 = case shown="True" w134 {
            tunnel: w133 -> [_ w210]
            tunnel: w64 -> [_ w206]
            frame False {
            }
            frame True {
              n88 = Unbundle By Name(w206) -> ("Main Screen.Depthz"=w208:refnum<vi>)
              n89 = property class="Bool (strict)"(reference=w208, "Value"=FALSE) -> (reference out=w207:refnum<vi>, error out=w209:errorcluster)  [unwired: 1 in]
              n90 = Close Reference(reference=w207, error in (no error)=w209) -> ()  [unwired: 1 out]
              "DepthZ" <- w210
            }
          }
          n91 = property class="WFChart (strict)"(reference=w156, "Value"=w147) -> (reference out=w154:refnum<vi>, error out=w155:errorcluster)  [unwired: 1 in]
          n92 = Unbundle By Name(w64) -> ("Main Screen.Time ( HH:MM:SS ) 2"=w84:refnum<vi>)
          n93 = Unbundle By Name(w64) -> ("Main Screen.Depth (µm)"=w130:refnum<vi>)
          n94 = property class="DigNum (strict)"(reference=w157, "Value"=w97) -> (reference out=w159:refnum<vi>, error out=w158:errorcluster)  [unwired: 1 in]
          n95 = call "ELAPSED TIMER VI FOR MONITOR Loop.vi"("TARGET"=w118, "RESET"=FALSE ("PAUSE"), "PAUSE"=w63) -> ("ELAPSED INDICATION"=w105:bool, "ELAPSED TIMER"=w83:dbl)  [unwired: 6 in, 1 out]
          n96 = Subtract(x=w133, y=w132) -> (x-y=w124:dbl)
          n97 = Multiply(x=w124, y=-1000.0) -> (x*y=w125:dbl)
          n98 = Close Reference(reference=w154, error in (no error)=w155) -> ()  [unwired: 1 out]
          n99 = property class="DigNum (strict)"(reference=w84, "Value"=w83) -> (reference out=w116:refnum<vi>, error out=w117:errorcluster)  [unwired: 1 in]
          n100 = Unbundle By Name(w64) -> ("Main Screen.WearGp"=w127:refnum<vi>)
          n101 = property class="DigNum (strict)"(reference=w130, "Value"=w125) -> (reference out=w131:refnum<vi>, error out=w129:errorcluster)  [unwired: 1 in]
          n102 = Close Reference(reference=w159, error in (no error)=w158) -> ()  [unwired: 1 out]
          n103 = property class="WFChart (strict)"(reference=w127, "Value"=w125) -> (reference out=w128:refnum<vi>, error out=w126:errorcluster)  [unwired: 1 in]
          n104 = Unbundle By Name(w64) -> ("Main Screen.Cyclic Friction Force (N)"=w101:refnum<vi>)
          n105 = Unbundle By Name(w64) -> ("Main Screen.Friction Force (N)"=w114:refnum<vi>)
          n106 = Close Reference(reference=w116, error in (no error)=w117) -> ()  [unwired: 1 out]
          n107 = Close Reference(reference=w131, error in (no error)=w129) -> ()  [unwired: 1 out]
          n108 = Unbundle By Name(w64) -> ("Main Screen.Speed (RPM)"=w73:refnum<vi>)
          n109 = Unbundle By Name(w64) -> ("Main Screen.speed mm/sec"=w75:refnum<vi>)
          n110 = Close Reference(reference=w128, error in (no error)=w126) -> ()  [unwired: 1 out]
          n111 = property class="DigNum (strict)"(reference=w73, "Value"=w70) -> (reference out=w71:refnum<vi>, error out=w72:errorcluster)  [unwired: 1 in]
          n112 = property class="WFChart (strict)"(reference=w75, "Value"=w74) -> (reference out=w77:refnum<vi>, error out=w76:errorcluster)  [unwired: 1 in]
          n113 = Unbundle By Name(w64) -> ("Main Screen.Load Disable Trip"=w67:refnum<vi>)
          n114 = property class="DigNum (strict)"(reference=w114) -> (reference out=w115:refnum<vi>, error out=w113:errorcluster, "Value"=w107:dbl)  [unwired: 1 in]
          n115 = property class="DigNum (strict)"(reference=w101) -> (reference out=w99:refnum<vi>, error out=w100:errorcluster, "Value"=w98:dbl)  [unwired: 1 in]
          n116 = Unbundle By Name(w64) -> ("Main Screen.Cyclic Friction Force (N) Graph"=w104:refnum<vi>)
          n117 = Unbundle By Name(w64) -> ("Motion Module.Scratch"=w82:refnum<vi>)
          n118 = Unbundle By Name(w64) -> ("Main Screen.Friction Force (N) Graph"=w85:refnum<vi>)
          n119 = property class="Bool (strict)"(reference=w67) -> (reference out=w69:refnum<vi>, error out=w68:errorcluster, "Value"=w66:bool)  [unwired: 1 in]
          n120 = property class="Bool (strict)"(reference=w82) -> (reference out=w91:refnum<vi>, error out=w92:errorcluster, "Value"=w90:bool)  [unwired: 1 in]
          n121 = Close Reference(reference=w71, error in (no error)=w72) -> ()  [unwired: 1 out]
          n122 = Close Reference(reference=w77, error in (no error)=w76) -> ()  [unwired: 1 out]
          n123 = Close Reference(reference=w115, error in (no error)=w113) -> ()  [unwired: 1 out]
          n124 = Close Reference(reference=w99, error in (no error)=w100) -> ()  [unwired: 1 out]
          n125 = Unbundle By Name(w64) -> ("Main Screen.NL disp 2"=w89:refnum<vi>)
          n126 = Close Reference(reference=w91, error in (no error)=w92) -> ()  [unwired: 1 out]
          n127 = Close Reference(reference=w69, error in (no error)=w68) -> ()  [unwired: 1 out]
          n128 = property class="WFChart (strict)"(reference=w104, "Value"=w98) -> (reference out=w102:refnum<vi>, error out=w103:errorcluster)  [unwired: 1 in]
          n129 = property class="WFChart (strict)"(reference=w85, "Value"=w107) -> (reference out=w111:refnum<vi>, error out=w112:errorcluster)  [unwired: 1 in]
          n130 = property class="DigNum (strict)"(reference=w89) -> (reference out=w87:refnum<vi>, error out=w88:errorcluster, "Value"=w86:dbl)  [unwired: 1 in]
          n131 = case shown="True" w105 {
            tunnel: w64 -> [_ w184]
            tunnel: w90 -> [_ w183]
            tunnel: w66 -> [_ w182]
            frame False {
              n132 = local write "Test Stop Temp"(FALSE ("Test Stop Temp")) -> ()
            }
            frame True {
              n133 = case shown="False" w182 {
                tunnel: w184 -> [w187 _]
                tunnel: w183 -> [w186 _]
                frame False {
                  n134 = case shown="False" w186 {
                    tunnel: w187 -> [w188 _]
                    frame False {
                      (unwired) FALSE ("y")
                      n135 = Unbundle By Name(w188) -> ("Main Screen.STOP"=w194:refnum<vi>)
                      n136 = Unbundle By Name(w188) -> ("Main Screen.Start Test"=w191:refnum<vi>)
                      n137 = Unbundle By Name(w188) -> ("Main Screen.Start Test Temp"=w202:refnum<vi>)
                      n138 = Unbundle By Name(w188) -> ("Main Screen.STOP"=w201:refnum<vi>)
                      n139 = property class="Bool (strict)"(reference=w194, "Visible"=FALSE) -> (reference out=w196:refnum<vi>, error out=w195:errorcluster)  [unwired: 1 in]
                      n140 = property class="Bool (strict)"(reference=w191, "Visible"=TRUE) -> (reference out=w189:refnum<vi>, error out=w190:errorcluster)  [unwired: 1 in]
                      n141 = property class="Bool (strict)"(reference=w202, "Value"=FALSE) -> (reference out=w204:refnum<vi>, error out=w203:errorcluster)  [unwired: 1 in]
                      n142 = property class="Bool (strict)"(reference=w201, "Value"=TRUE) -> (reference out=w199:refnum<vi>, error out=w200:errorcluster)  [unwired: 1 in]
                      n143 = Close Reference(reference=w196, error in (no error)=w195) -> ()  [unwired: 1 out]
                      n144 = Close Reference(reference=w189, error in (no error)=w190) -> ()  [unwired: 1 out]
                      n145 = Close Reference(reference=w204, error in (no error)=w203) -> ()  [unwired: 1 out]
                      n146 = Close Reference(reference=w199, error in (no error)=w200) -> ()  [unwired: 1 out]
                    }
                    frame True {
                    }
                  }
                }
                frame True {
                }
              }
              "Test Stop Temp" <- TRUE ("Test Stop Temp")
            }
          }
          n147 = Close Reference(reference=w111, error in (no error)=w112) -> ()  [unwired: 1 out]
          n148 = Close Reference(reference=w102, error in (no error)=w103) -> ()  [unwired: 1 out]
          n149 = Unbundle By Name(w64) -> ("Main Screen.Cyclic Coefficient of Friction"=w95:refnum<vi>)
          n150 = Close Reference(reference=w87, error in (no error)=w88) -> ()  [unwired: 1 out]
          n151 = Unbundle By Name(w64) -> ("Main Screen.Coefficient of Friction"=w109:refnum<vi>)
          n152 = Divide(x=w98, y=w86) -> (x/y=w94:dbl)
          n153 = Divide(x=w107, y=w86) -> (x/y=w106:dbl)
          n154 = property class="WFChart (strict)"(reference=w109, "Value"=w106) -> (reference out=w110:refnum<vi>, error out=w108:errorcluster)  [unwired: 1 in]
          n155 = property class="WFChart (strict)"(reference=w95, "Value"=w94) -> (reference out=w93:refnum<vi>, error out=w96:errorcluster)  [unwired: 1 in]
          n156 = Close Reference(reference=w110, error in (no error)=w108) -> ()  [unwired: 1 out]
          n157 = Close Reference(reference=w93, error in (no error)=w96) -> ()  [unwired: 1 out]
        }
      }
    }
    frame Error {
    }
  }
